vi "Init Hardware.vi"(8 "error in (no error)":errorcluster, 11 "MFLI Driver in":refnum<class "MFLI Driver.lvclass">) -> (0 "error out":errorcluster, 3 "MFLI Driver out":refnum<class "MFLI Driver.lvclass">)   [LabVIEW 2021, in "MFLI Driver.lvclass"]
uses:
  MFLI Driver.lvclass
  C:/github/NHMFL_Core/Libraries/Instruments/Instrument Driver/Instrument Driver.lvclass
  Instrument Driver/Instrument Driver.lvclass/Instrument Driver.ctl
  Instrument Driver/Read Recorder name.vi
  Instrument Driver/Write Channel names.vi
  Instrument Driver/Write Channel units.vi
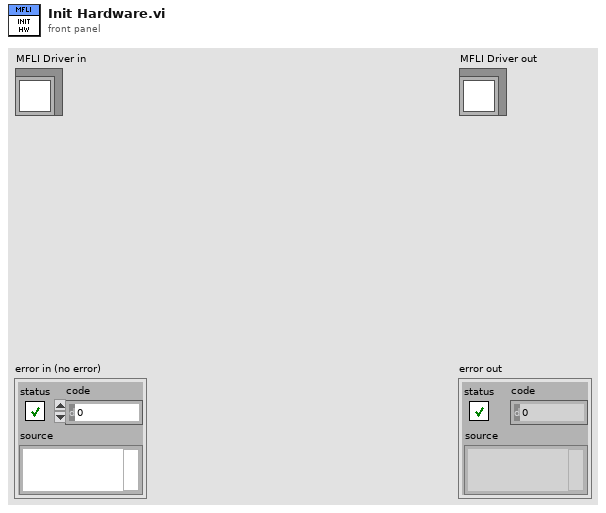
[diagram p1: front panel]
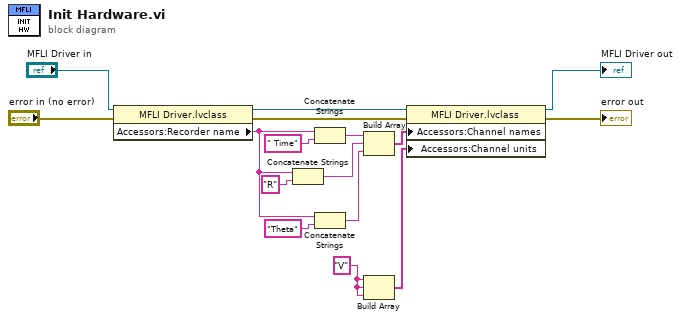
[diagram p0: block diagram]
diagram:
  w4 = "V"
  n1 = property class="MFLI Driver.lvclass"(reference="MFLI Driver in", error in="error in (no error)") -> (reference out=w15:refnum<class "MFLI Driver.lvclass">, error out=w16:errorcluster, "Accessors:Recorder name"=w6:string)
  n2 = Concatenate Strings(w6, "R") -> (w10:string)
  n3 = Concatenate Strings(w6, " Time") -> (w12:string)
  n4 = Concatenate Strings(w6, "Theta") -> (w5:string)
  n5 = Build Array(w12, w10, w5) -> (w14:string[])
  n6 = Build Array(w4, w4, w4) -> (w3:string[])
  n7 = property class="MFLI Driver.lvclass"(reference=w15, error in=w16, "Accessors:Channel names"=w14, "Accessors:Channel units"=w3) -> (reference out=→"MFLI Driver out":refnum<class "MFLI Driver.lvclass">, error out=→"error out":errorcluster)
